vi "display_and_capture_pattern.vi"(6 "#Phase Shifts":i32, 7 "capture images ?":bool, 9 "intial phase shift":dbl, 10 "#fringes":dbl, 11 "Camera ID":T1 caption="Session In") -> ()   [LabVIEW 2011]
uses:
  <vilib>/userDefined/High Color/IMAQdx.ctl
  global_vars.vi
  <vilib>/vision/driver/NI_Vision_Acquisition_Software.lvlib
  <vilib>/vision/NI_Vision_Development_Module.lvlib
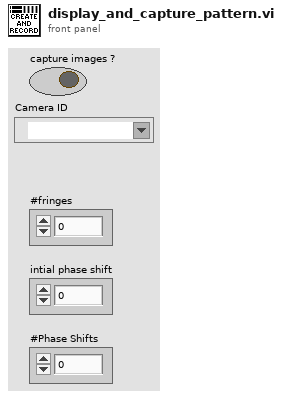
[diagram p1: front panel]
types:
  T1 = typedef "IMAQdx.ctl" = refnum<k21>
  T2 = typedef "IMAQ Image.ctl" = refnum<image>
  T3 = typedef "Image Type" = u32
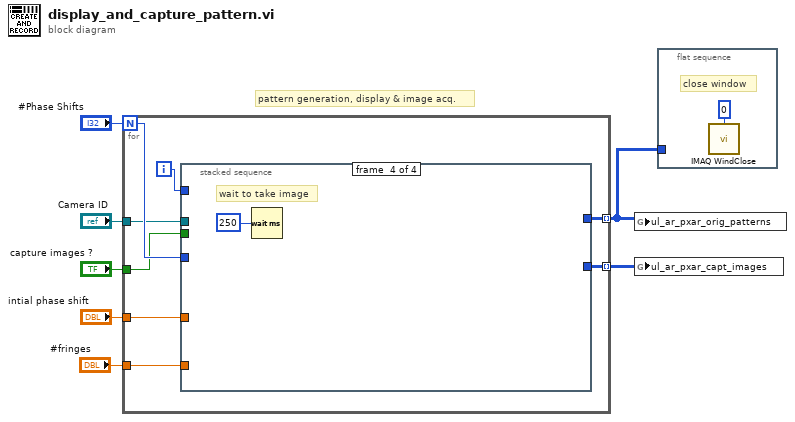
[diagram p0: block diagram]
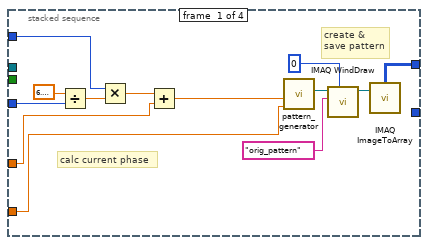
[diagram p2: hidden frame]
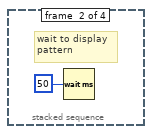
[diagram p3: hidden frame]
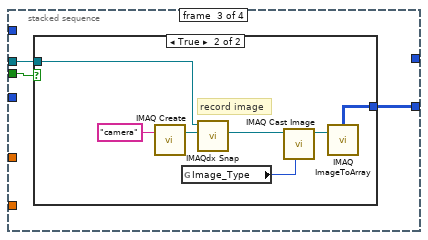
[diagram p4: hidden frame]
diagram:
  # "pattern generation, display & image acq."
  n1 = for {
    N: "#Phase Shifts" -> [w13]
    tunnel: [w15] -> w1 mode=indexing
    tunnel: [w14] -> w2 mode=indexing
    tunnel: "#fringes" -> [w11]
    tunnel: "intial phase shift" -> [w10]
    tunnel: "capture images ?" -> [w9]
    tunnel: "Camera ID" -> [w8]
    i -> [w12]
    n2 = stacked-sequence {
      tunnel: w13 -> [w19 _ _ _]
      tunnel: [w24 _ _ _] -> w15
      tunnel: [_ _ w32 _] -> w14
      tunnel: w12 -> [w20 _ _ _]
      tunnel: w11 -> [w17 _ _ _]
      tunnel: w10 -> [w16 _ _ _]
      tunnel: w9 -> [_ _ w31 _]
      tunnel: w8 -> [_ _ w30 _]
      frame #0 {
        # "calc current phase"
        # "create & \nsave pattern"
        n3 = Divide(x=6.283185307179586, y=w19) -> (x/y=w22:dbl)
        n4 = Multiply(x=w20, y=w22) -> (x*y=w21:dbl)
        n5 = Add(x=w21, y=w16) -> (x+y=w18:dbl)
        n6 = call "pattern_generator.vi"("fringe number"=w17, "phase"=w18) -> ("fringe pattern"=w26:T2)  [unwired: 8 in, 1 out]
        n7 = call "IMAQ WindDraw"("Window Number (0...15)"=0, "Title"="orig_pattern", "Image"=w26) -> ("Image Out (duplicate)"=w25:T2)  [unwired: 7 in, 1 out]
        n8 = call "IMAQ ImageToArray"("Image"=w25) -> ("Image Pixels (U8)"=w24:u8[][])  [unwired: 3 in, 4 out]
      }
      frame #1 {
        # "wait to display \npattern"
        n9 = Wait (ms)(milliseconds to wait=u32 50) -> ()  [unwired: 1 out]
      }
      frame #2 {
        n10 = case shown="True" w31 {
          tunnel: [_ w34] -> w32
          tunnel: w30 -> [_ w33]
          frame False {
          }
          frame True {
            # "record image"
            n11 = call "IMAQ Create"("Image Name"="camera") -> ("New Image"=w39:T2)  [unwired: 3 in, 2 out]
            n12 = global read "global_vars.vi" "Image_Type"() -> (w35:T3)
            n13 = call <vilib>:"IMAQdx Snap.vi"("Image In"=w39, "Session In"=w33) -> ("Image Out"=w37:T2)  [unwired: 7 in, 2 out]
            n14 = call "IMAQ Cast Image"("Image Type"=w35, "Image Src"=w37) -> ("Image Dst Out"=w36:T2)  [unwired: 8 in, 1 out]
            n15 = call "IMAQ ImageToArray"("Image"=w36) -> ("Image Pixels (U8)"=w34:u8[][])  [unwired: 3 in, 4 out]
          }
        }
      }
      frame #3 {
        # "wait to take image"
        n16 = Wait (ms)(milliseconds to wait=u32 250) -> ()  [unwired: 1 out]
      }
    }
  }
  n17 = global write "global_vars.vi" "ul_ar_pxar_orig_patterns"(w1) -> ()
  n18 = global write "global_vars.vi" "ul_ar_pxar_capt_images"(w2) -> ()
  n19 = flat-sequence {
    tunnel: w1 -> [_]
    frame #0 {
      # "close window"
      n20 = call "IMAQ WindClose"("Window Number (0...15)"=0) -> ()  [unwired: 5 in, 1 out]
    }
  }
